vi "VendingMachine Main.vi"() -> ()   [LabVIEW 2020]
doc: "This VI is simple demonstrator of vending machine based on state machine structure. Program was created for the LabVIEW tutorial needs. Comments in Polish language."
uses:
  Ctrls/StateEnum.ctl
panel:
  out "Cash":string="0"
  in  "Pizza":bool
  in  "Chips":bool
  in  "ColaCan":bool
  in  "Cola":bool
  in  "Error In":errorcluster
  in  "Deposit":bool
  in  "stop":bool
  # "Icons made by Freepick (https://www.freepik.com) from Flaticon (https://www.flaticon.com/)"
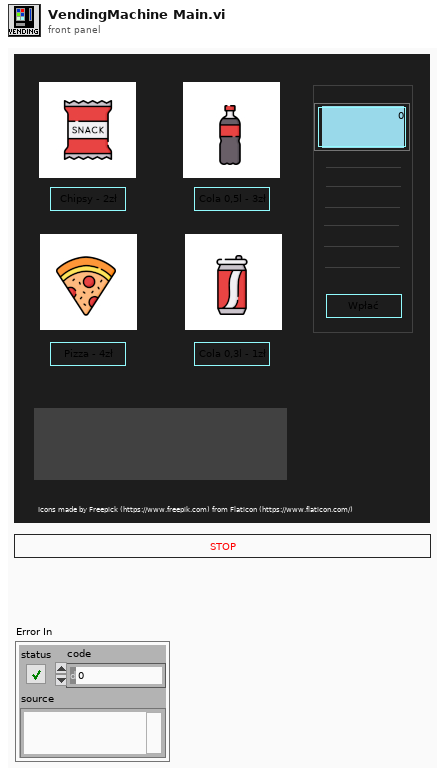
[diagram p1: front panel]
types:
  T1 = typedef "StateEnum.ctl" = enum16{"IDLE", "INSERT MONEY", "SELECTION", "DISPENSE"}
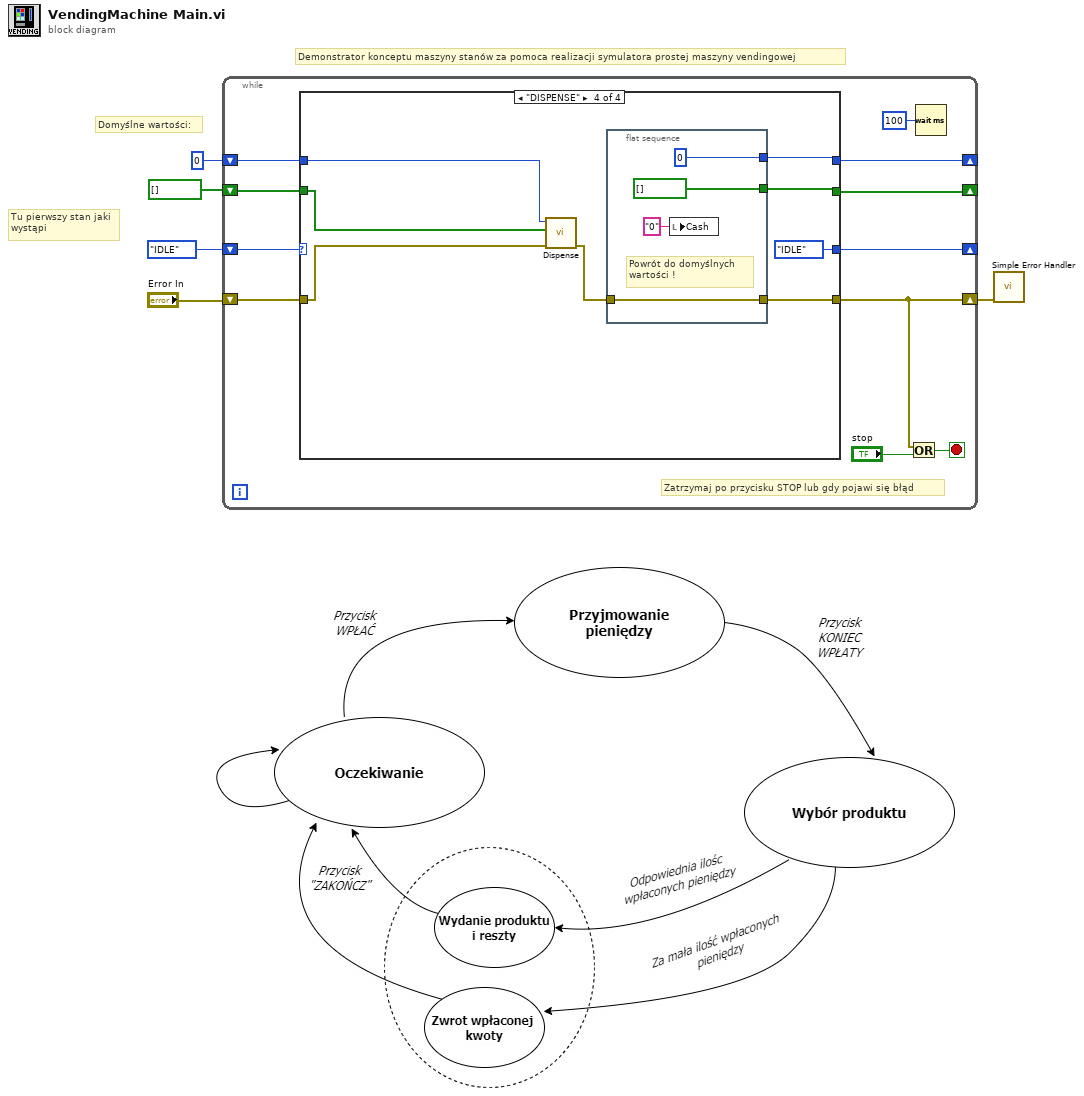
[diagram p0: block diagram]
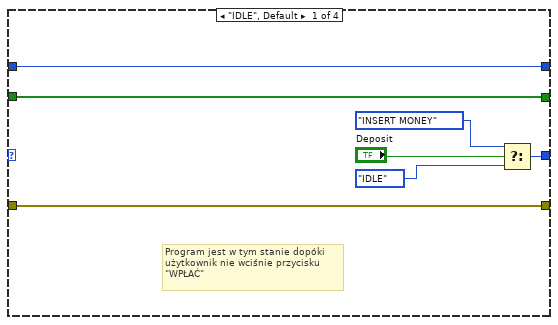
[diagram p2: hidden frame]
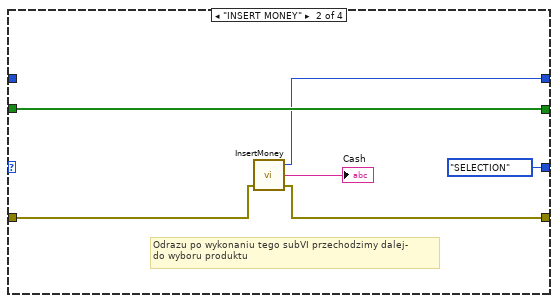
[diagram p3: hidden frame]
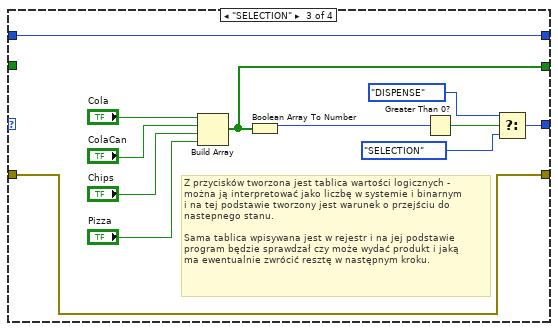
[diagram p4: hidden frame]
diagram:
  # "Tu pierwszy stan jaki\nwystąpi"
  # "Domyślne wartości:"
  # "Demonstrator konceptu maszyny stanów za pomoca realizacji symulatora prostej maszyny vendingowej"
  n1 = while {
    shift-right: [w14] -> _
    shift-left: StateEnum."IDLE" -> [w15]
    shift-right: [w11] -> w1
    shift-left: "Error In" -> [w13]
    shift-right: [w9] -> _
    shift-left: 0 -> [w10]
    shift-right: [w7] -> _
    shift-left: bool[] [] -> [w8]
    stop <- w12 stop-if-true
    # "Zatrzymaj po przycisku STOP lub gdy pojawi się błąd"
    n2 = case shown="\"DISPENSE\"" w15 {
      tunnel: [w20 StateEnum."SELECTION" w31 StateEnum."IDLE"] -> w14
      tunnel: w13 -> [w19 w28 w30 w48]
      tunnel: [w19 w27 w30 w44] -> w11
      tunnel: w10 -> [w18 _ w41 w47]
      tunnel: [w18 w24 w41 w42] -> w9
      tunnel: w8 -> [w17 w26 _ w46]
      tunnel: [w17 w26 w32 w43] -> w7
      frame "IDLE", Default {
        # "Program jest w tym stanie dopóki\nużytkownik nie wciśnie przycisku \n\"WPŁAĆ\""
        n3 = Select(t=StateEnum."INSERT MONEY", s="Deposit", f=StateEnum."IDLE") -> (s? t:f=w20:T1)
      }
      frame "INSERT MONEY" {
        # "Odrazu po wykonaniu tego subVI przechodzimy dalej-\ndo wyboru produktu"
        n4 = call "InsertMoney.vi"("Error In"=w28) -> ("Error Out"=w27:errorcluster, "InsertMoney"=→"Cash":string, "InsertsMoney"=w24:i32)  [unwired: 2 in]
      }
      frame "SELECTION" {
        # "Z przycisków tworzona jest tablica wartości logicznych -\nmożna ją interpretować jako liczbę w systemie i binarnym\ni na tej podstawie tworzony jest warunek o przejściu do \nnastepnego stanu.\n\nSama tablica wpisywana jest w rejestr i na jej podstawie \nprogram będzie sprawdzał czy może wydać produkt i jaką \nma ewentualnie zwrócić resztę w następnym kroku."
        n5 = Build Array("Cola", "ColaCan", "Chips", "Pizza") -> (w32:bool[])
        n6 = Boolean Array To Number(Boolean array=w32) -> (number=w36:u32)
        n7 = Greater Than 0?(x=w36) -> (x > 0?=w35:bool)
        n8 = Select(t=StateEnum."DISPENSE", s=w35, f=StateEnum."SELECTION") -> (s? t:f=w31:T1)
      }
      frame "DISPENSE" {
        n9 = call "Dispense.vi"("Error In"=w48, "Selection"=w46, "Money"=w47) -> ("Error Out"=w45:errorcluster)  [unwired: 8 in]
        n10 = flat-sequence {
          tunnel: w45 -> [w53]
          tunnel: [w53] -> w44
          tunnel: [bool[] []] -> w43
          tunnel: [0 ("InsertsMoney")] -> w42
          frame #0 {
            # "Powrót do domyślnych\nwartości !"
            n11 = local write "Cash"("0" ("Cash")) -> ()
          }
        }
      }
    }
    n12 = Or(x=w11, y="stop") -> (x .or. y?=w12:bool)
    n13 = Wait (ms)(milliseconds to wait=u32 100) -> ()  [unwired: 1 out]
  }
  n14 = call <vilib>:"Simple Error Handler.vi"("error in (no error)"=w1) -> ()  [unwired: 4 in, 5 out]
